vi "mWADC_DATA Record.vi"(7 "Direction":enum32{"CW", "CCW"}(radio), 8 "Record_Stop":bool, 9 "Angle per increment":dbl=100.0, 10 "MW_ADC":refnum<visa-resource-name>, 11 "MW motor":refnum<visa-resource-name>) -> (0 "error out":errorcluster, 1 "Data Recording":bool, 4 "Negetive_L":bool, 5 "Positive_L":bool)   [LabVIEW 2019]
uses:
  <vilib>/Utility/file.llb/Write Delimited Spreadsheet (DBL).vi
panel:
  out "Current possition (Revolutions)":dbl(knob) caption="Current Angle" scale=0.0..4.0
  out "Horizontal Progress Bar":i32(slide) scale=0.0..32768.0
  in  "Record_Start":bool
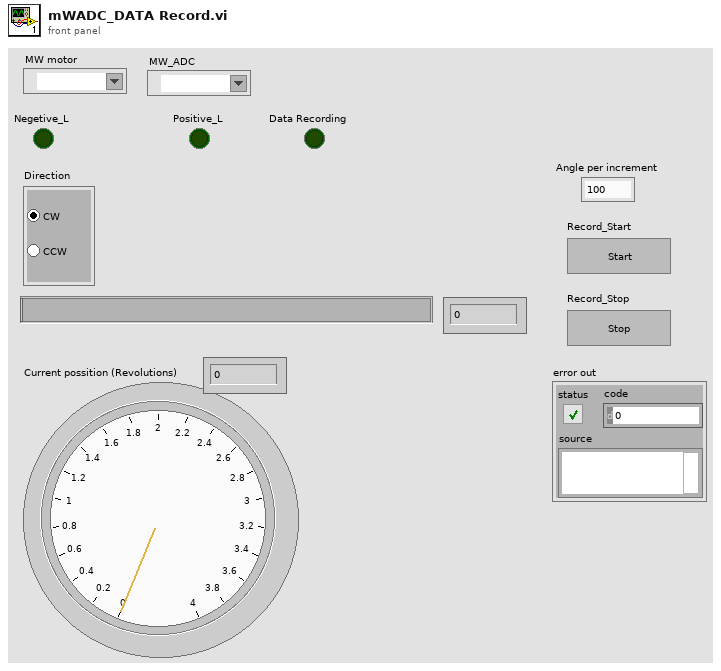
[diagram p1: front panel]
types:
  T1 = enum16{"open", "replace", "create", "open or create", "replace or create", "replace or create with confirmation"}
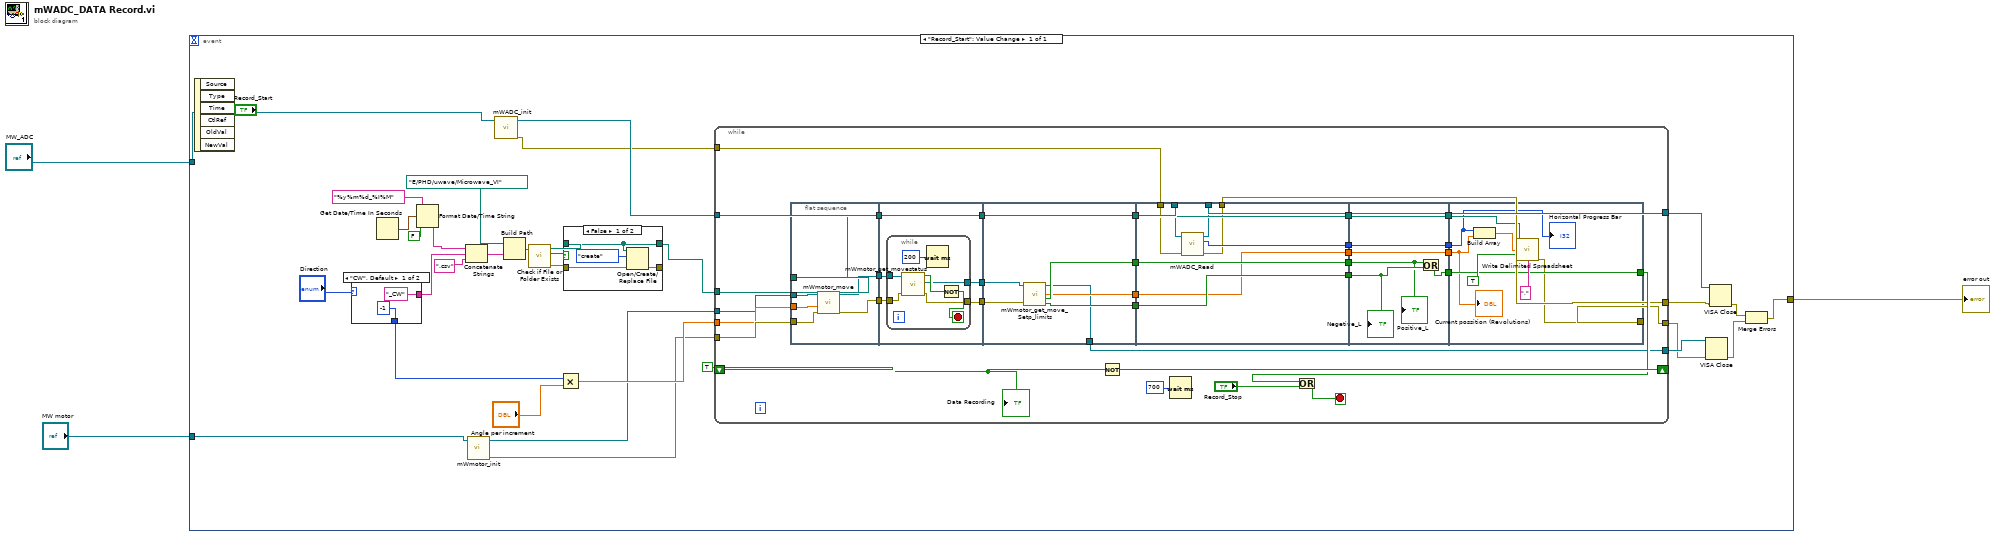
[diagram p0: block diagram]
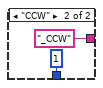
[diagram p2: hidden frame]
diagram:
  n1 = event shown="[0] \"Record_Start\": Value Change" {
    selector: _ -> [_]
    dyn-events: _ -> [_]
    timeout: _ -> [_]
    tunnel: "MW_ADC" -> [w16]
    tunnel: "MW motor" -> [w14]
    tunnel: [w4] -> w1
    event "Record_Start": Value Change {
      n2 = event-data() -> ()  [unwired: 1 in, 6 out]
      n3 = case shown="\"CW\", Default" "Direction" {
        tunnel: ["_CW" ("string") "_CCW" ("string")] -> w23
        tunnel: [-1 ("x") 1 ("x")] -> w21
        frame "CW", Default {
        }
        frame "CCW" {
        }
      }
      n4 = Get Date/Time In Seconds() -> (seconds since 1Jan1904=w27:timestamp)
      n5 = Format Date/Time String(time format string (%c)="%y%m%d_%I%M", seconds (now)=w27, UTC format=FALSE) -> (date/time string=w24:string)
      n6 = Concatenate Strings(w24, w23, ".csv" ("string")) -> (w33:string)
      n7 = call "mWmotor_init.vi"("mWMotor_Port"=w14) -> ("error out"=w11:errorcluster, "reference out"=w13:refnum<visa-resource-name>)  [unwired: 9 in]
      n8 = call "mWADC_init.vi"("mWADC_Port"=w16) -> ("error out"=w12:errorcluster, "reference out"=w15:refnum<visa-resource-name>)  [unwired: 9 in]
      n9 = Build Path(base path=path "E:/PHD/uwave/Microwave_VI" ("path"), name or relative path=w33) -> (appended path=w32:path)
      n10 = call <vilib>:"Check if File or Folder Exists.vi"("path"=w32) -> ("error out"=w30:errorcluster, "file or folder exists?"=w29:bool, "dup path"=w31:path)  [unwired: 8 in]
      n11 = Multiply(x=w21, y="Angle per increment") -> (x*y=w17:dbl)
      n12 = case shown="False" w29 {
        tunnel: w31 -> [w123 w126]
        tunnel: [w124 w127] -> _
        tunnel: [w123 w126] -> w18
        tunnel: w30 -> [w122 w127]
        frame False {
          n13 = Open/Create/Replace File(file path (use dialog)=w123, error in=w122, operation (0:open)=T1."create") -> (error out=w124:errorcluster)  [unwired: 3 in, 2 out]
        }
        frame True {
        }
      }
      n14 = while {
        shift-right: [w69] -> _
        shift-left: TRUE ("x") -> [w68]
        tunnel: w18 -> [w65]
        tunnel: w11 -> [w66]
        tunnel: [w35] -> w7
        tunnel: w15 -> [w51]
        tunnel: [w41] -> w10
        tunnel: w17 -> [w40]
        tunnel: w13 -> [w39]
        tunnel: [w38] -> w9
        tunnel: w12 -> [w37]
        tunnel: [w36] -> w8
        stop <- w60 stop-if-true
        n15 = flat-sequence {
          tunnel: w66 -> [w74]
          tunnel: w65 -> [w75]
          tunnel: [w75] -> w62
          tunnel: [w73] -> w54
          tunnel: [w72] -> w53
          tunnel: w40 -> [w71]
          tunnel: w39 -> [w70]
          tunnel: [w80] -> w64
          tunnel: w62 -> [w79]
          tunnel: [w79] -> w61
          tunnel: w54 -> [w78]
          tunnel: w53 -> [w77]
          tunnel: [w76] -> w52
          tunnel: w64 -> [w93]
          tunnel: w61 -> [w94]
          tunnel: [w94] -> w59
          tunnel: w52 -> [w92]
          tunnel: [w91] -> w49
          tunnel: [w90] -> w47
          tunnel: [w89] -> w43
          tunnel: [w88] -> w38
          tunnel: w59 -> [w103]
          tunnel: [w103] -> w58
          tunnel: w51 -> [w102]
          tunnel: [w101] -> w50
          tunnel: w49 -> [w101]
          tunnel: [w100] -> w48
          tunnel: w47 -> [w100]
          tunnel: [w99] -> w45
          tunnel: [w98] -> w44
          tunnel: w43 -> [w98]
          tunnel: [w97] -> w41
          tunnel: w37 -> [w96]
          tunnel: [w95] -> w36
          tunnel: w58 -> [w109]
          tunnel: [w109] -> w57
          tunnel: [w108] -> w56
          tunnel: w50 -> [w107]
          tunnel: w48 -> [w106]
          tunnel: [w105] -> w46
          tunnel: w45 -> [w105]
          tunnel: w44 -> [w104]
          tunnel: [w104] -> w42
          tunnel: w57 -> [w117]
          tunnel: w56 -> [w114]
          tunnel: [w114] -> w55
          tunnel: w46 -> [w110]
          tunnel: w42 -> [w111]
          tunnel: [w112] -> w35
          frame #0 {
            n16 = call "mWmotor_move.vi"("error in (no error)"=w74, "Degrees To move"=w71, "MW motor"=w70) -> ("error out"=w73:errorcluster, "VISA resource name out"=w72:refnum<visa-resource-name>)  [unwired: 7 in]
          }
          frame #1 {
            n17 = while {
              tunnel: [w83] -> w80
              tunnel: w78 -> [w85]
              tunnel: w77 -> [w82]
              tunnel: [w81] -> w76
              stop <- w86 stop-if-true
              n18 = call "mWmotor_get_movestatus.vi"("error in (no error)"=w85, "VISA resource name"=w82) -> ("error out"=w83:errorcluster, "VISA resource name out"=w81:refnum<visa-resource-name>, "Boolean"=w84:bool)  [unwired: 7 in]
              n19 = Wait (ms)(milliseconds to wait=u32 200) -> ()  [unwired: 1 out]
              n20 = Not(x=w84) -> (.not. x?=w86:bool)
            }
          }
          frame #2 {
            n21 = call "mWmotor_get_move_Setp_limits.vi"("VISA resource name"=w92, "error in (no error)"=w93) -> ("VISA resource name out"=w88:refnum<visa-resource-name>, "Revolutions"=w89:dbl, "Positive_L"=w90:bool, "Negetive_L"=w91:bool)  [unwired: 7 in, 3 out]
          }
          frame #3 {
            n22 = call "mWADC_Read.vi"("error in (no error)"=w96, "MW_ADC"=w102) -> ("error out"=w95:errorcluster, "ADC Count"=w99:i32, "VISA resource name out"=w97:refnum<visa-resource-name>)  [unwired: 7 in]
          }
          frame #4 {
            n23 = Or(x=w106, y=w107) -> (x .or. y?=w108:bool)
            "Positive_L" <- w106
            "Negetive_L" <- w107
          }
          frame #5 {
            n24 = Build Array(w110, w111) -> (w113:dbl[])
            n25 = call-poly <vilib>:"Write Delimited Spreadsheet.vi"("file path (dialog if empty)"=w117, "1D data"=w113, "append to file? (new file:F)"=TRUE, "delimiter (\\t)"="," ("delimiter (\\t)")) -> ("error out"=w112:errorcluster)  [unwired: 10 in, 1 out]
            "Current possition (Revolutions)" <- w111
            "Horizontal Progress Bar" <- w110
          }
        }
        n26 = Not(x=w68) -> (.not. x?=w69:bool)
        n27 = Wait (ms)(milliseconds to wait=u32 700) -> ()  [unwired: 1 out]
        n28 = Or(x=w55, y="Record_Stop") -> (x .or. y?=w60:bool)
        "Data Recording" <- w68
      }
      n29 = VISA Close(VISA resource name=w9, error in (no error)=w7) -> (error out=w6:errorcluster)
      n30 = VISA Close(VISA resource name=w10, error in (no error)=w8) -> (error out=w5:errorcluster)
      n31 = Merge Errors(w5, w6) -> (w4:errorcluster)
    }
  }
  "error out" <- w1
